vi "Zad4_kolokwium.vi"() -> ()   [LabVIEW 2012]
panel:
  out "Wartość rezystancji":string
  in  "wartość natężenia prądu":dbl
  in  "Wartość napięcia prądu":dbl
  # "Program oblicza rezystancję na podstawie podanego napięcia i natężenia prądu"
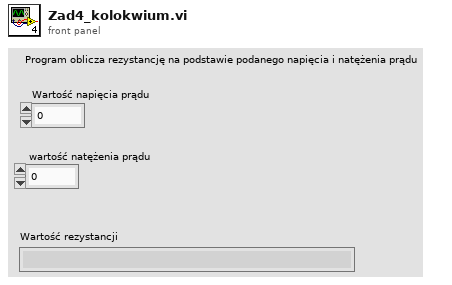
[diagram p1: front panel]
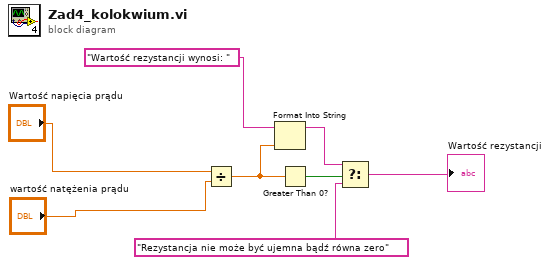
[diagram p0: block diagram]
diagram:
  n1 = Divide(x="Wartość napięcia prądu", y="wartość natężenia prądu") -> (x/y=w3:dbl)
  n2 = Format Into String(initial string="Wartość rezystancji wynosi: ", w3) -> (resulting string=w4:string)  [unwired: 2 in, 1 out]
  n3 = Greater Than 0?(x=w3) -> (x > 0?=w6:bool)
  n4 = Select(t=w4, s=w6, f="Rezystancja nie może być ujemna bądź równa zero") -> (s? t:f=→"Wartość rezystancji":string)
